vi "Replace Slashes.vi"(11 "time stamp":timestamp) -> (3 "Date & Time String":string)   [LabVIEW 2020]
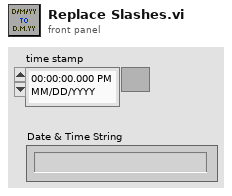
[diagram p1: front panel]
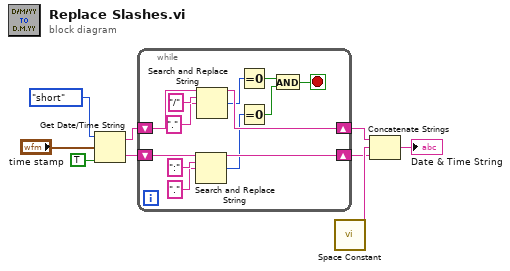
[diagram p0: block diagram]
diagram:
  n1 = Get Date/Time String(date format (0)=enum16{"short", "long", "abbreviated"}."short", seconds (now)="time stamp", want seconds? (F)=TRUE) -> (date string=w8:string, time string=w7:string)
  n2 = while {
    shift-right: [w22] -> w4
    shift-left: w8 -> [w18]
    shift-right: [w16] -> w3
    shift-left: w7 -> [w17]
    stop <- w11 stop-if-true
    n3 = Search and Replace String(input string=w17, search string=":", replace string="." ("replace string (\"\")")) -> (result string=w16:string, number of replacements=w13:i32)  [unwired: 5 in, 2 out]
    n4 = Search and Replace String(input string=w18, search string="/", replace string="." ("replace string (\"\")")) -> (result string=w22:string, number of replacements=w19:i32)  [unwired: 5 in, 2 out]
    n5 = Equal To 0?(x=w19) -> (x = 0?=w10:bool)
    n6 = Equal To 0?(x=w13) -> (x = 0?=w12:bool)
    n7 = And(x=w10, y=w12) -> (x .and. y?=w11:bool)
  }
  n8 = call <vilib>:"Space Constant.vi"() -> ("String"=w5:string)
  n9 = Concatenate Strings(w4, w5, w3) -> (→"Date & Time String":string)
